vi "Whisker stim 2.vi"() -> ()   [LabVIEW 2020]
uses:
  <vilib>/MakerHub/LINX/Private/Type Defs/LINX Ref.ctl
  <vilib>/MakerHub/LINX/Private/Type Defs/Platform.ctl
  <vilib>/MakerHub/LINX/Private/Type Defs/Interface.ctl
  <vilib>/MakerHub/LINX/Private/Device/Type Defs/LINX Device Config.ctl
  <vilib>/MakerHub/LINX/Private/Device/Type Defs/TCP Config.ctl
  <vilib>/MakerHub/LINX/Private/Device/Type Defs/Channels.ctl
  <vilib>/MakerHub/LINX/Public/Peripherals/Digital/Digital Write 1 Chan.vi
  <vilib>/MakerHub/LINX/Public/Peripherals/Digital/Digital Write N Chans.vi
  <vilib>/MakerHub/LINX/Private/Local IO/LinxDigitalWrite.vi
  <vilib>/MakerHub/LINX/Public/Utilities/Check Channel.vi
  <vilib>/MakerHub/LINX/Private/Utilties/Generate Error.vi
  <vilib>/MakerHub/LINX/Public/Sensors/Motion/Servo/Servo Set Pulse Width One Channel.vi
  <vilib>/MakerHub/LINX/Public/Sensors/Motion/Servo/Servo.lvlib
  <vilib>/MakerHub/LINX/LMH-LINX.lvlib
  <vilib>/MakerHub/LINX/Private/Device/Device.lvlib
panel:
  out "Suggested P2 time (s)":dbl
  out "Seq. iteration":i32
  in  "Wheel coupled":bool
  out "Speed plot":dbl(graph)
  in  "Steps/s":u32=1000
  in  "Steps to move":dbl
  in  "Direction":bool
  in  "Stop Stepper":bool=TRUE
  in  "Start stepper":bool=TRUE caption="Start"
  in  "Direction 2":enum16{"CLW", "CCLW", "Off"}(ring)
  in  "Direction":enum16{"CLW", "CCLW", "Off"}(ring)
  in  "Speed(Steps/s) 2":u32
  in  "Speed(Steps/s)":u32
  out "Spin iteration":i32
  in  "Spin Time 2 (s)":u32
  in  "Spin n loop":i32=1
  in  "Spin Time 1 (s)":u32=5
  in  "Time(s) off":u32
  in  "Mode":enum16{"Automatic", "Manual", "Wheel"}(ring)
  out "Stop":bool
  out "Active":bool
  in  "Pole move (Pulse Width, microS)":dbl(slide)=1000.0 scale=1000.0..2000.0
  out "LINX Resource":T1
  in  "Seq loop":i32=1
  in  "Current State":string
  # "Linear Actuator"
  # "`"
  # "Stepper Motor"
  # "Auto"
  # "Manual"
  # "Wheel coupled"
  # "0 = infinite"
  # "CLW"
  # "CCLW"
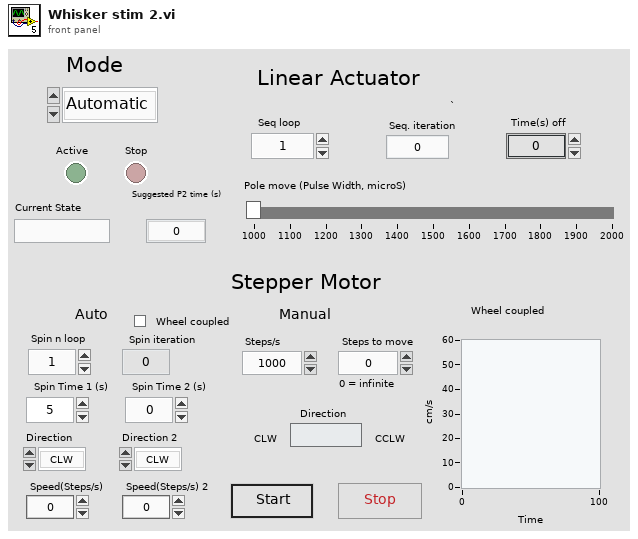
[diagram p1: front panel]
types:
  T1 = typedef "LMH-LINX.lvlib/LINX Ref.ctl" = cluster{"IO":T2, "Interface":T3, "LINX Device Config":T4}
  T2 = typedef "LMH-LINX.lvlib/Platform.ctl" = enum16{"Remote", "Local"}
  T3 = typedef "LMH-LINX.lvlib/Interface.ctl" = enum16{"Serial", "TCP"}
  T4 = typedef "LMH-LINX.lvlib/Device.lvlib/LINX Device Config.ctl" = cluster{"Interface":T3, "COM Port":refnum<visa-resource-name>, "TCP Configuration":T5, "Device Family":u8, "Device ID":u8, "Device Name":string, "TCP Ref":refnum<k5>, "Channels":T6}
  T5 = typedef "LMH-LINX.lvlib/Device.lvlib/TCP Config.ctl" = cluster{"IP Address":string, "Port":u16}
  T6 = typedef "LMH-LINX.lvlib/Channels.ctl" = cluster{"DI":u8[], "DO":u8[], "AI":u8[], "AO":u8[], "PWM":u8[], "QE":u8[], "UART":u8[], "I2C 2":u8[], "SPI":u8[], "CAN":u8[], "Servo":u8[], "AI Ref (V)":dbl, "AI Resolution (Bits)":u8, "AO Ref (V)":dbl, "AO Resolution (Bits)":u8}
  T7 = enum8{"Enabled", "Disabled", "Disabled and Grayed Out"}
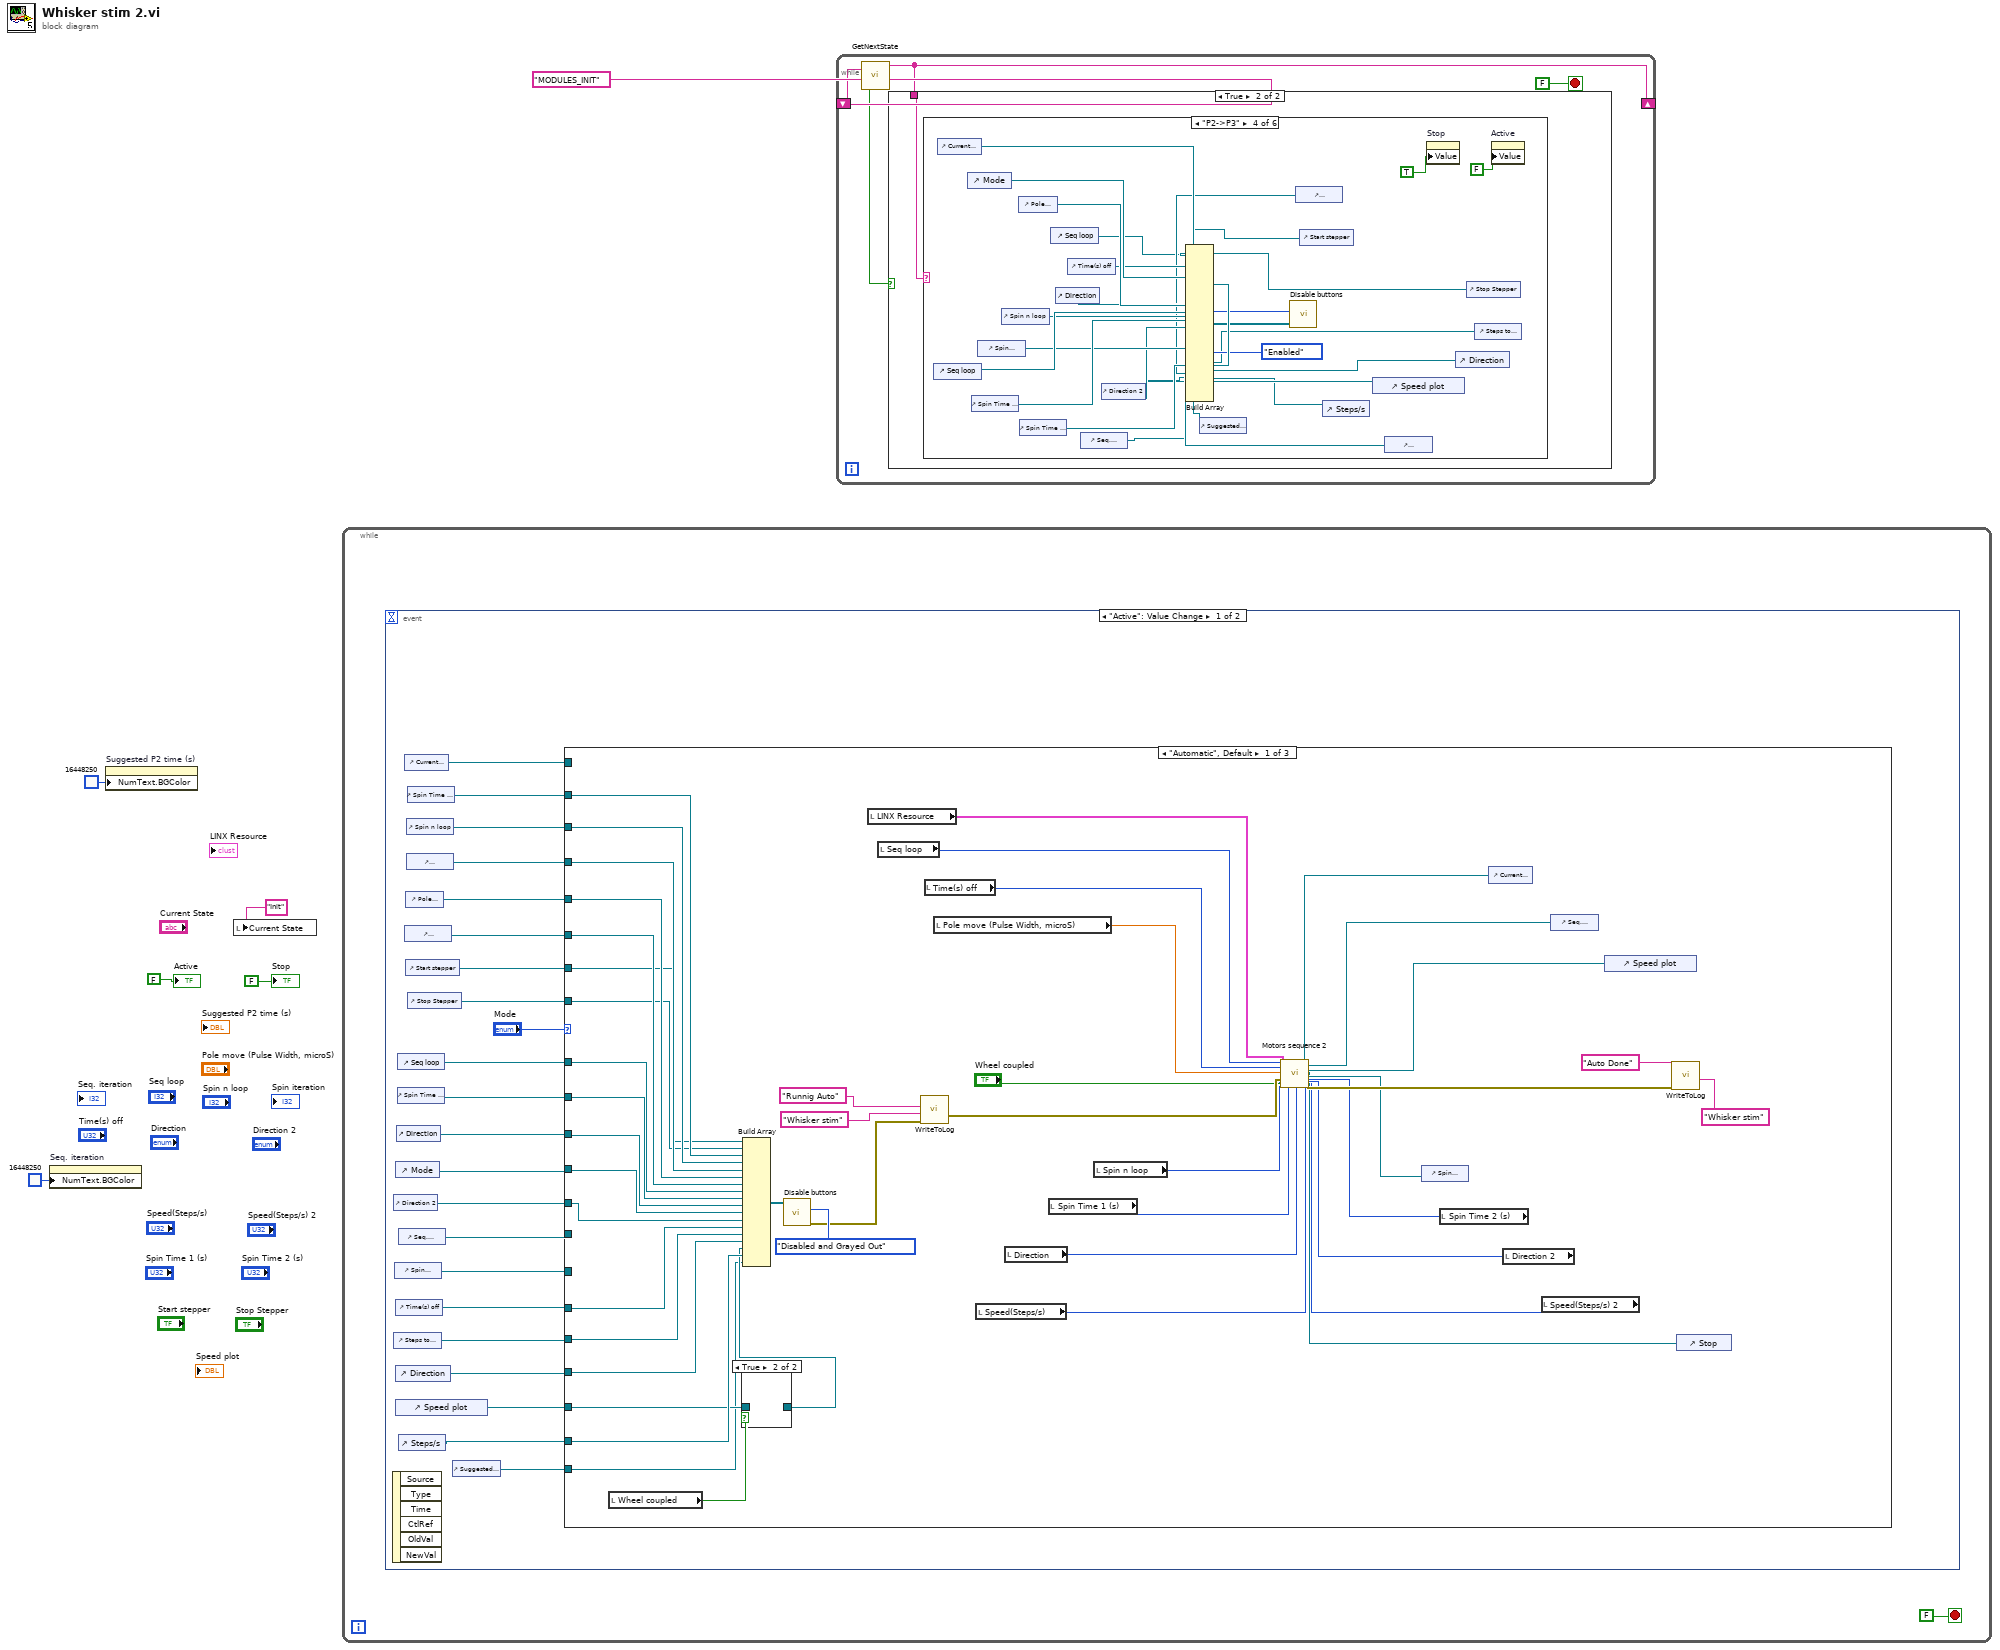
[diagram p0: block diagram]
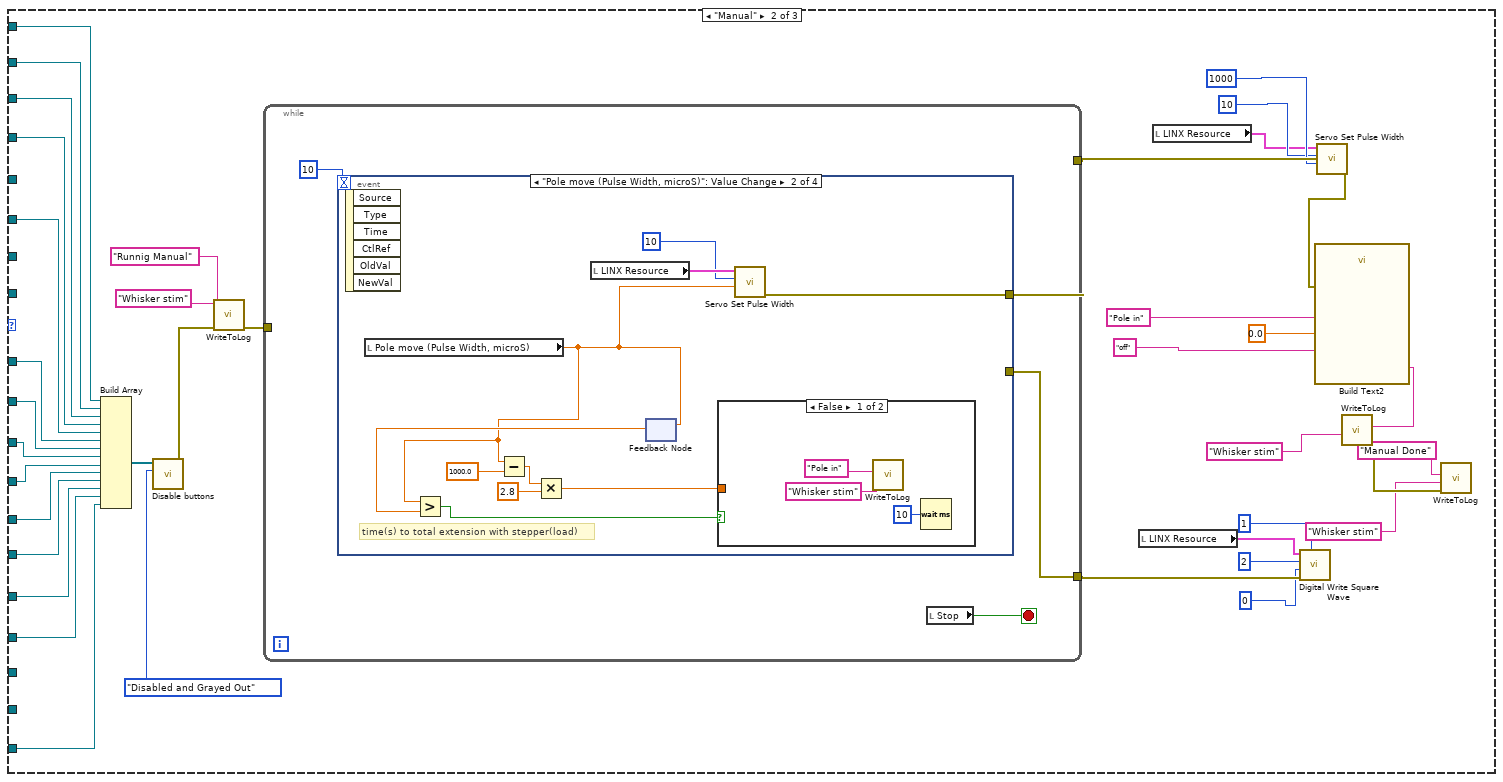
[diagram p3: hidden frame]
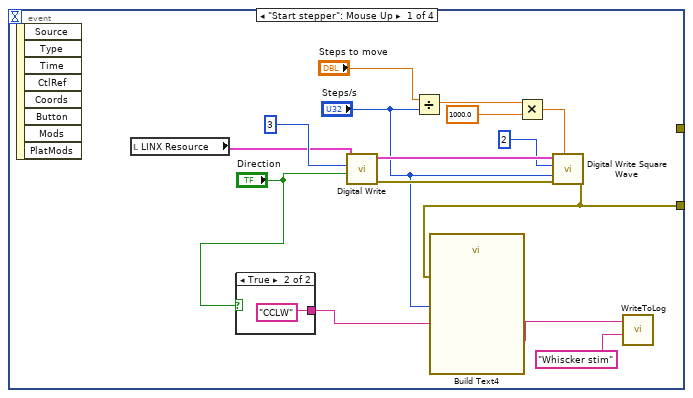
[diagram p4: hidden frame]
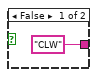
[diagram p5: hidden frame]
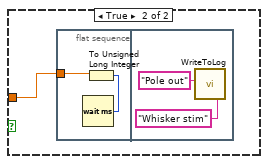
[diagram p6: hidden frame]
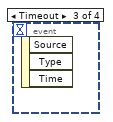
[diagram p7: hidden frame]
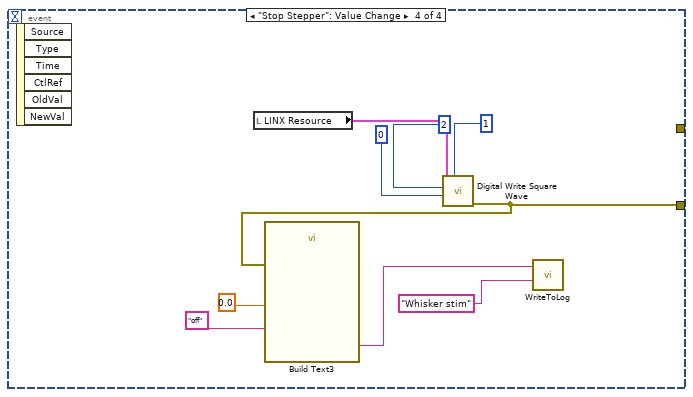
[diagram p8: hidden frame]
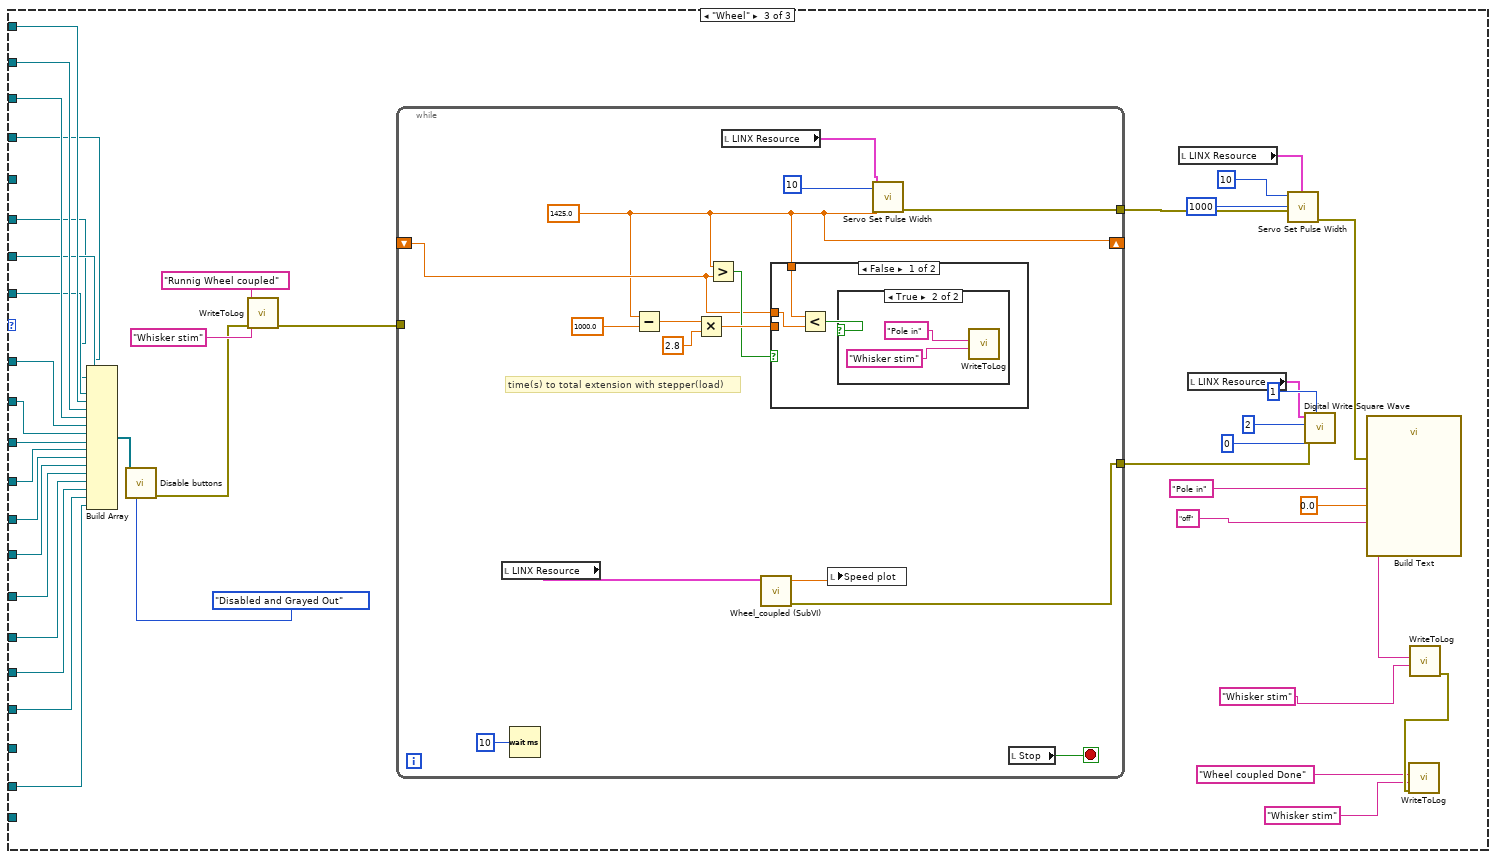
[diagram p9: hidden frame]
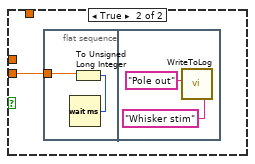
[diagram p11: hidden frame]
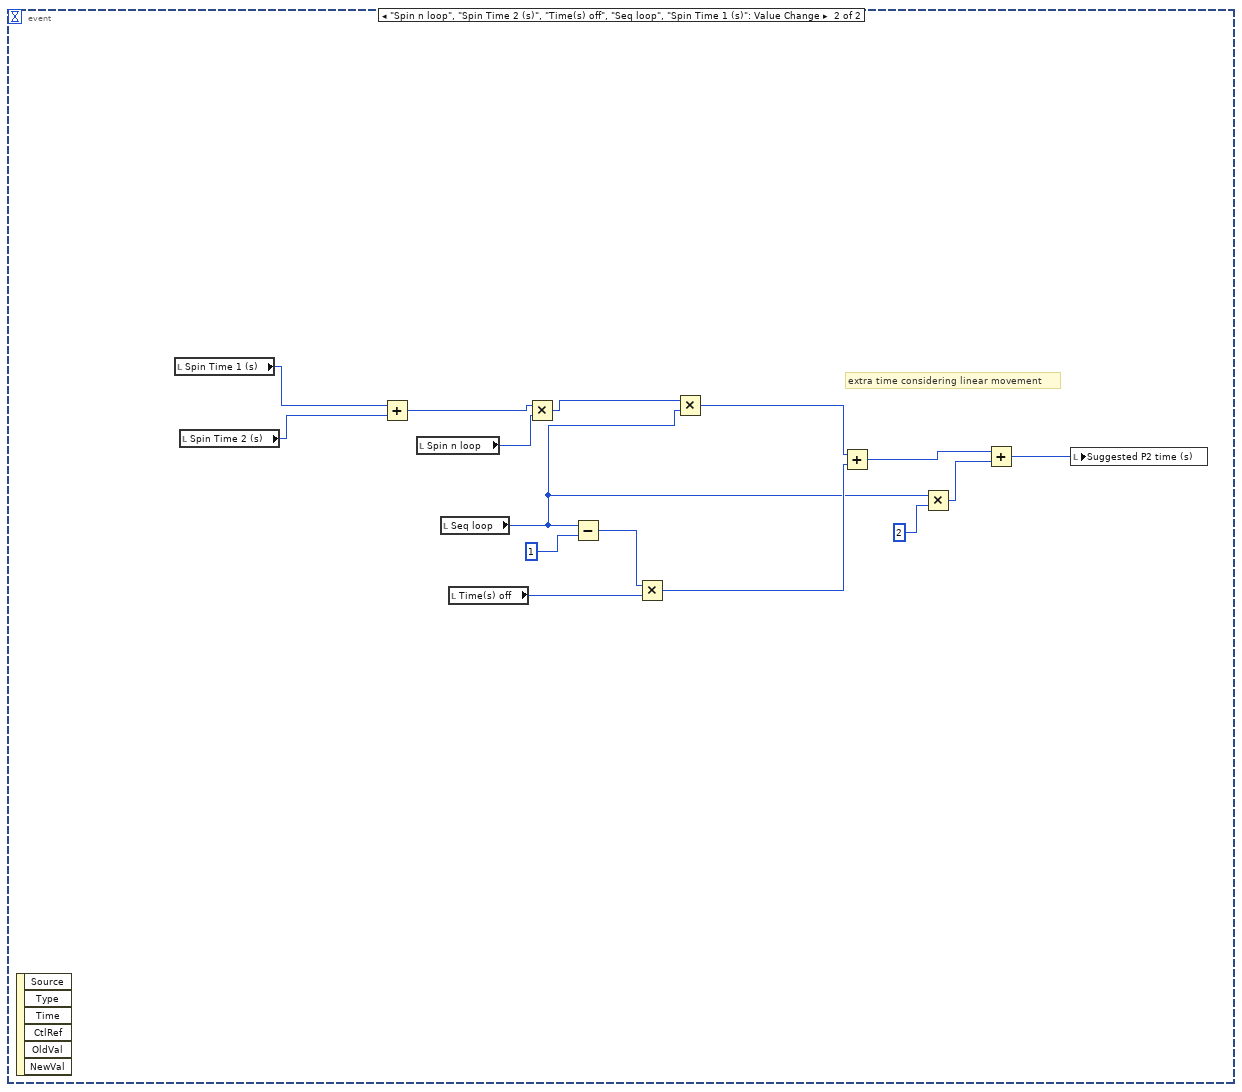
[diagram p12: hidden frame]
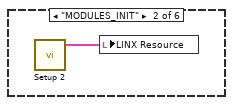
[diagram p15: hidden frame]
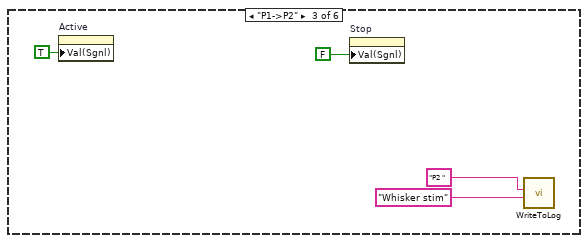
[diagram p16: hidden frame]
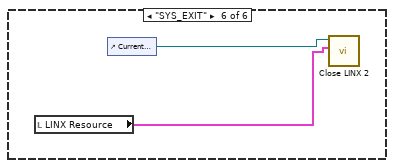
[diagram p18: hidden frame]
diagram:
  n1 = property on="Seq. iteration" class="DigNum (strict)"("NumText.BGColor"=u32 16448250 ("Numeric Text.Colors:BG Color")) -> ()  [unwired: 2 in, 2 out]
  n2 = property on="Suggested P2 time (s)" class="DigNum (strict)"("NumText.BGColor"=u32 16448250 ("Numeric Text.Text Colors:BG Color")) -> ()  [unwired: 2 in, 2 out]
  n3 = local write "Current State"("Init" ("State name")) -> ()
  n4 = while {
    stop <- FALSE stop-if-true
    n5 = event shown="[0] \"Active\": Value Change" {
      selector: _ -> [_ _]
      dyn-events: _ -> [_ _]
      timeout: _ -> [_ _]
      event "Active": Value Change {
        n6 = event-data() -> ()  [unwired: 1 in, 6 out]
        n7 = control-ref of="Direction 2"() -> (w20:refnum<vi>)
        n8 = control-ref of="Steps to move"() -> (w15:refnum<vi>)
        n9 = control-ref of="Spin iteration"() -> (w24:refnum<vi>)
        n10 = control-ref of="Mode"() -> (w25:refnum<vi>)
        n11 = control-ref of="Time(s) off"() -> (w16:refnum<vi>)
        n12 = control-ref of="Direction"() -> (w14:refnum<vi>)
        n13 = control-ref of="Speed plot"() -> (w13:refnum<vi>)
        n14 = control-ref of="Direction"() -> (w21:refnum<vi>)
        n15 = control-ref of="Seq loop"() -> (w29:refnum<vi>)
        n16 = control-ref of="Spin Time 1 (s)"() -> (w23:refnum<vi>)
        n17 = control-ref of="Seq. iteration"() -> (w9:refnum<vi>)
        n18 = control-ref of="Steps/s"() -> (w10:refnum<vi>)
        n19 = control-ref of="Current State"() -> (w22:refnum<vi>)
        n20 = control-ref of="Speed(Steps/s) 2"() -> (w18:refnum<vi>)
        n21 = control-ref of="Pole move (Pulse Width, microS)"() -> (w28:refnum<vi>)
        n22 = control-ref of="Start stepper"() -> (w12:refnum<vi>)
        n23 = control-ref of="Spin n loop"() -> (w27:refnum<vi>)
        n24 = control-ref of="Speed(Steps/s)"() -> (w19:refnum<vi>)
        n25 = control-ref of="Spin Time 2 (s)"() -> (w26:refnum<vi>)
        n26 = control-ref of="Stop Stepper"() -> (w11:refnum<vi>)
        n27 = control-ref of="Suggested P2 time (s)"() -> (w8:refnum<vi>)
        n28 = case shown="\"Automatic\", Default" "Mode" {
          tunnel: w26 -> [w73 w82 w180]
          tunnel: w27 -> [w72 w81 w179]
          tunnel: w28 -> [w70 _ _]
          tunnel: w29 -> [w68 w78 w178]
          tunnel: w21 -> [w74 w89 w176]
          tunnel: w25 -> [w75 w88 w175]
          tunnel: w20 -> [w62 w87 w174]
          tunnel: w24 -> [_ w85 w172]
          tunnel: w19 -> [w71 w80 w163]
          tunnel: w23 -> [w65 w90 w177]
          tunnel: w22 -> [_ w83 w181]
          tunnel: w18 -> [w69 w79 w164]
          tunnel: w16 -> [w67 w84 w171]
          tunnel: w9 -> [_ w86 w173]
          tunnel: w15 -> [w66 _ w170]
          tunnel: w14 -> [w64 _ w169]
          tunnel: w13 -> [w53 w77 _]
          tunnel: w10 -> [w63 _ w168]
          tunnel: w12 -> [w61 _ w166]
          tunnel: w11 -> [w60 _ w167]
          tunnel: w8 -> [w30 _ _]
          frame "Automatic", Default {
            n29 = local read "Wheel coupled"() -> (w54:bool)
            n30 = case shown="True" w54 {
              tunnel: w53 -> [w76 _]
              tunnel: [w76 _] -> w52
              frame False {
              }
              frame True {
              }
            }
            n31 = Build Array(w61, w60, w73, w72, w71, w70, w69, w68, w65, w74, w75, w62, w67, w66, w64, w52, w63, w30) -> (w59:refnum<vi>[])
            n32 = call "Disable buttons.vi"("Disabled"=T7."Disabled and Grayed Out", "Array"=w59) -> ("error out"=w55:errorcluster)  [unwired: 9 in]
            n33 = local read "LINX Resource"() -> (w47:T1)
            n34 = local read "Seq loop"() -> (w38:i32)
            n35 = call "WriteToLog.vi"("error in (no error)"=w55, "Category"="Whisker stim", "Message"="Runnig Auto") -> ("error out"=w51:errorcluster)  [unwired: 8 in]
            n36 = local read "Time(s) off"() -> (w31:u32)
            n37 = local read "Pole move (Pulse Width, microS)"() -> (w45:dbl)
            n38 = local read "Speed(Steps/s)"() -> (w44:u32)
            n39 = local read "Direction"() -> (w41:enum16{"CLW", "CCLW", "Off"})
            n40 = local read "Spin Time 1 (s)"() -> (w43:u32)
            n41 = local read "Spin n loop"() -> (w35:i32)
            n42 = control-ref of="Spin iteration"() -> (w33:refnum<vi>)
            n43 = local read "Spin Time 2 (s)"() -> (w42:u32)
            n44 = control-ref of="Current State"() -> (w46:refnum<vi>)
            n45 = local read "Direction 2"() -> (w40:enum16{"CLW", "CCLW", "Off"})
            n46 = local read "Speed(Steps/s) 2"() -> (w36:u32)
            n47 = control-ref of="Seq. iteration"() -> (w34:refnum<vi>)
            n48 = control-ref of="Speed plot"() -> (w37:refnum<vi>)
            n49 = control-ref of="Stop"() -> (w32:refnum<vi>)
            n50 = call "Motors sequence 2.vi"("LINX Resource"=w47, "Current State"=w46, "Pole move(microS)"=w45, "Speed(Steps/s)"=w44, "Error In"=w51, "Wheel"="Wheel coupled", "Spin time/Rest(1)"=w43, "Spin n loops"=w35, "Spin time(2)"=w42, "Speed(Steps/s) 2"=w36, "Direction"=w41, "Pole ms to wait off"=w31, "Direction 2"=w40, "Seq. iteration 2"=w34, "Stop"=w32, "Speed plot 2"=w37, "Seq. loop"=w38, "Spin iteration 2"=w33) -> ("error out"=w48:errorcluster)  [unwired: 8 in, 1 out]
            n51 = call "WriteToLog.vi"("error in (no error)"=w48, "Category"="Whisker stim", "Message"="Auto Done") -> ()  [unwired: 8 in, 1 out]
          }
          frame "Manual" {
            n52 = Build Array(w83, w82, w81, w80, w79, w78, w90, w89, w88, w87, w86, w85, w84, w77) -> (w91:refnum<vi>[])
            n53 = call "Disable buttons.vi"("Disabled"=T7."Disabled and Grayed Out", "Array"=w91) -> ("error out"=w97:errorcluster)  [unwired: 9 in]
            n54 = call "WriteToLog.vi"("error in (no error)"=w97, "Category"="Whisker stim", "Message"="Runnig Manual") -> ("error out"=w96:errorcluster)  [unwired: 8 in]
            n55 = while {
              tunnel: [w116] -> w113
              tunnel: [w115] -> w110
              tunnel: w96 -> [_]
              stop <- w118 stop-if-true
              n56 = event shown="[1] \"Pole move (Pulse Width, microS)\": Value Change" {
                selector: _ -> [_ _ _ _]
                dyn-events: _ -> [_ _ _ _]
                timeout: 10 -> [_ _ _ _]
                tunnel: [_ w143 _ _] -> w116
                tunnel: [w122 _ _ w154] -> w115
                event "Start stepper": Mouse Up {
                  n57 = event-data() -> ()  [unwired: 1 in, 8 out]
                  n58 = local read "LINX Resource"() -> (w126:T1)
                  n59 = case shown="True" "Direction" {
                    tunnel: ["CLW" "CCLW"] -> w120
                    frame False {
                    }
                    frame True {
                    }
                  }
                  n60 = call-poly <vilib>:"Digital Write.vi"("Output Value"="Direction", "DO Channel"=u8 3, "LINX Resource"=w126) -> ("Error Out"=w123:errorcluster, "LINX Resource"=w130:T1)  [unwired: 7 in]
                  n61 = Divide(x="Steps to move", y="Steps/s") -> (x/y=w128:dbl)
                  n62 = Multiply(x=w128, y=1000.0) -> (x*y=w132:dbl)
                  n63 = call <vilib>:"Digital Write Square Wave.vi"("Duration (ms)"=w132, "Error In"=w123, "Frequency (Hz)"="Steps/s", "Channel"=u8 2, "LINX Resource"=w130) -> ("Error Out"=w122:errorcluster)  [unwired: 5 in, 1 out]
                  n64 = call "Build Text4"("speed"="Steps/s", "spinmode"=w120, "error in (no error)"=w122) -> ("Result"=w124:string)  [unwired: 11 in, 1 out]
                  n65 = call "WriteToLog.vi"("Category"="Whiscker stim", "Message"=w124) -> ()  [unwired: 9 in, 1 out]
                }
                event "Pole move (Pulse Width, microS)": Value Change {
                  # "time(s) to total extension with stepper(load)"
                  n66 = event-data() -> ()  [unwired: 1 in, 6 out]
                  n67 = local read "Pole move (Pulse Width, microS)"() -> (w136:dbl)
                  n68 = Subtract(x=w136, y=1000.0) -> (x-y=w142:dbl)
                  n69 = Multiply(x=w142, y=2.8) -> (x*y=w139:dbl)
                  n70 = local read "LINX Resource"() -> (w145:T1)
                  n71 = feedback #1() -> (w137:dbl)  [unwired: 1 in]
                  n72 = Greater?(x=w136, y=w137) -> (0:w138:bool)
                  n73 = feedback-in #1(w136) -> ()
                  n74 = case shown="False" w138 {
                    tunnel: w139 -> [_ w149]
                    frame False {
                      n75 = call "WriteToLog.vi"("Category"="Whisker stim", "Message"="Pole in") -> ()  [unwired: 9 in, 1 out]
                      n76 = Wait (ms)(milliseconds to wait=u32 10) -> ()  [unwired: 1 out]
                    }
                    frame True {
                      n77 = flat-sequence {
                        tunnel: w149 -> [w150]
                        frame #0 {
                          n78 = To Unsigned Long Integer(number=w150) -> (unsigned 32bit integer=w151:u32)
                          n79 = Wait (ms)(milliseconds to wait=w151) -> ()  [unwired: 1 out]
                        }
                        frame #1 {
                          n80 = call "WriteToLog.vi"("Category"="Whisker stim", "Message"="Pole out") -> ()  [unwired: 9 in, 1 out]
                        }
                      }
                    }
                  }
                  n81 = call-poly <vilib>:"Servo Set Pulse Width.vi"("Pulse Width (uS)"=w136, "Servo Channel"=u8 10, "LINX Resource"=w145) -> ("Error Out"=w143:errorcluster)  [unwired: 7 in, 1 out]
                }
                event Timeout {
                  n82 = event-data() -> ()  [unwired: 1 in, 3 out]
                }
                event "Stop Stepper": Value Change {
                  n83 = event-data() -> ()  [unwired: 1 in, 6 out]
                  n84 = local read "LINX Resource"() -> (w159:T1)
                  n85 = call <vilib>:"Digital Write Square Wave.vi"("Duration (ms)"=u32 1, "Frequency (Hz)"=u32 0, "Channel"=u8 2, "LINX Resource"=w159) -> ("Error Out"=w154:errorcluster)  [unwired: 6 in, 1 out]
                  n86 = call "Build Text3"("speed"=0.0, "spinmode"="off", "error in (no error)"=w154) -> ("Result"=w156:string)  [unwired: 11 in, 1 out]
                  n87 = call "WriteToLog.vi"("Category"="Whisker stim", "Message"=w156) -> ()  [unwired: 9 in, 1 out]
                }
              }
              n88 = local read "Stop"() -> (w118:bool)
            }
            n89 = local read "LINX Resource"() -> (w105:T1)
            n90 = local read "LINX Resource"() -> (w106:T1)
            n91 = call <vilib>:"Digital Write Square Wave.vi"("Duration (ms)"=u32 1, "Error In"=w110, "Frequency (Hz)"=u32 0, "Channel"=u8 2, "LINX Resource"=w105) -> ()  [unwired: 5 in, 2 out]
            n92 = call-poly <vilib>:"Servo Set Pulse Width.vi"("Error In"=w113, "Pulse Width (uS)"=u16 1000, "Servo Channel"=u8 10, "LINX Resource"=w106) -> ("Error Out"=w98:errorcluster)  [unwired: 6 in, 1 out]
            n93 = call "Build Text2"("speed"=0.0, "spinmode"="off", "step"="Pole in", "error in (no error)"=w98) -> ("Result"=w102:string)  [unwired: 10 in, 1 out]
            n94 = call "WriteToLog.vi"("Category"="Whisker stim", "Message"=w102) -> ("error out"=w94:errorcluster)  [unwired: 9 in]
            n95 = call "WriteToLog.vi"("error in (no error)"=w94, "Category"="Whisker stim", "Message"="Manual Done") -> ()  [unwired: 8 in, 1 out]
          }
          frame "Wheel" {
            n96 = Build Array(w163, w164, w166, w167, w181, w180, w179, w178, w177, w176, w175, w174, w173, w172, w171, w170, w169, w168) -> (w165:refnum<vi>[])
            n97 = call "Disable buttons.vi"("Disabled"=T7."Disabled and Grayed Out", "Array"=w165) -> ("error out"=w185:errorcluster)  [unwired: 9 in]
            n98 = call "WriteToLog.vi"("error in (no error)"=w185, "Category"="Whisker stim", "Message"="Runnig Wheel coupled") -> ("error out"=w186:errorcluster)  [unwired: 8 in]
            n99 = while {
              tunnel: [w217] -> w204
              tunnel: [w213] -> w197
              shift-right: [w206] -> _
              shift-left: _ -> [w207]
              tunnel: w186 -> [_]
              stop <- w219 stop-if-true
              w206 = 1425.0 ("Pole move (Pulse Width, microS)")
              # "time(s) to total extension with stepper(load)"
              n100 = local read "LINX Resource"() -> (w218:T1)
              n101 = Wait (ms)(milliseconds to wait=u32 10) -> ()  [unwired: 1 out]
              n102 = Subtract(x=w206, y=1000.0) -> (x-y=w211:dbl)
              n103 = Multiply(x=w211, y=2.8) -> (x*y=w209:dbl)
              n104 = Greater?(x=w206, y=w207) -> (0:w208:bool)
              n105 = local read "LINX Resource"() -> (w215:T1)
              n106 = call "Wheel_coupled (SubVI).vi"("LINX Resource"=w218) -> ("error out"=w217:errorcluster, "Speed plot"=w205:dbl)  [unwired: 9 in]
              n107 = case shown="False" w208 {
                tunnel: w209 -> [_ w225]
                tunnel: w206 -> [w222 _]
                tunnel: w207 -> [w221 _]
                frame False {
                  n108 = Less?(x=w222, y=w221) -> (x < y?=w220:bool)
                  n109 = case shown="True" w220 {
                    frame False {
                    }
                    frame True {
                      n110 = call "WriteToLog.vi"("Category"="Whisker stim", "Message"="Pole in") -> ()  [unwired: 9 in, 1 out]
                    }
                  }
                }
                frame True {
                  n111 = flat-sequence {
                    tunnel: w225 -> [w226]
                    frame #0 {
                      n112 = To Unsigned Long Integer(number=w226) -> (unsigned 32bit integer=w227:u32)
                      n113 = Wait (ms)(milliseconds to wait=w227) -> ()  [unwired: 1 out]
                    }
                    frame #1 {
                      n114 = call "WriteToLog.vi"("Category"="Whisker stim", "Message"="Pole out") -> ()  [unwired: 9 in, 1 out]
                    }
                  }
                }
              }
              n115 = local write "Speed plot"(w205) -> ()
              n116 = call-poly <vilib>:"Servo Set Pulse Width.vi"("Pulse Width (uS)"=w206, "Servo Channel"=u8 10, "LINX Resource"=w215) -> ("Error Out"=w213:errorcluster)  [unwired: 7 in, 1 out]
              n117 = local read "Stop"() -> (w219:bool)
            }
            n118 = local read "LINX Resource"() -> (w198:T1)
            n119 = local read "LINX Resource"() -> (w201:T1)
            n120 = call-poly <vilib>:"Servo Set Pulse Width.vi"("Error In"=w197, "Pulse Width (uS)"=u16 1000, "Servo Channel"=u8 10, "LINX Resource"=w198) -> ("Error Out"=w188:errorcluster)  [unwired: 6 in, 1 out]
            n121 = call <vilib>:"Digital Write Square Wave.vi"("Duration (ms)"=u32 1, "Error In"=w204, "Frequency (Hz)"=u32 0, "Channel"=u8 2, "LINX Resource"=w201) -> ()  [unwired: 5 in, 2 out]
            n122 = call "Build Text"("speed"=0.0, "spinmode"="off", "step"="Pole in", "error in (no error)"=w188) -> ("Result"=w190:string)  [unwired: 10 in, 1 out]
            n123 = call "WriteToLog.vi"("Category"="Whisker stim", "Message"=w190) -> ("error out"=w184:errorcluster)  [unwired: 9 in]
            n124 = call "WriteToLog.vi"("error in (no error)"=w184, "Category"="Whisker stim", "Message"="Wheel coupled Done") -> ()  [unwired: 8 in, 1 out]
          }
        }
      }
      event "Spin n loop", "Spin Time 2 (s)", "Time(s) off", "Seq loop", "Spin Time 1 (s)": Value Change {
        # "extra time considering linear movement"
        n125 = event-data() -> ()  [unwired: 1 in, 6 out]
        n126 = local read "Spin Time 1 (s)"() -> (w243:u32)
        n127 = local read "Spin Time 2 (s)"() -> (w244:u32)
        n128 = Add(x=w243, y=w244) -> (x+y=w242:u32)
        n129 = local read "Spin n loop"() -> (w241:i32)
        n130 = local read "Seq loop"() -> (w233:i32)
        n131 = local read "Time(s) off"() -> (w239:u32)
        n132 = Multiply(x=w242, y=w241) -> (x*y=w240:u32)
        n133 = Subtract(x=w233, y=1) -> (x-y=w237:i32)
        n134 = Multiply(x=w237, y=w239) -> (x*y=w235:u32)
        n135 = Multiply(x=w240, y=w233) -> (x*y=w236:u32)
        n136 = Add(x=w236, y=w235) -> (x+y=w234:u32)
        n137 = Multiply(x=w233, y=2) -> (x*y=w231:i32)
        n138 = Add(x=w234, y=w231) -> (x+y=w230:u32)
        n139 = local write "Suggested P2 time (s)"(w230) -> ()
      }
    }
  }
  n140 = while {
    shift-right: [w245] -> _
    shift-left: "MODULES_INIT" ("Next state") -> [w247]
    stop <- FALSE stop-if-true
    n141 = call "GetNextState.vi"("Current state"=w247) -> ("State has changed?"=w246:bool, "Next state"=w245:string)  [unwired: 9 in]
    n142 = case shown="True" w246 {
      tunnel: w245 -> [_ w249]
      frame False {
      }
      frame True {
        n143 = case shown="\"P2->P3\"" w249 {
          frame "False", Default {
          }
          frame "MODULES_INIT" {
            n144 = call "Setup 2.vi"() -> ("LINX Resource"=w250:T1)  [unwired: 10 in, 1 out]
            n145 = local write "LINX Resource"(w250) -> ()
          }
          frame "P1->P2" {
            n146 = property on="Active" class="Bool (strict)"("Val(Sgnl)"=TRUE ("Value (Signaling)")) -> ()  [unwired: 2 in, 2 out]
            n147 = property on="Stop" class="Bool (strict)"("Val(Sgnl)"=FALSE ("Value (Signaling)")) -> ()  [unwired: 2 in, 2 out]
            n148 = call "WriteToLog.vi"("Category"="Whisker stim", "Message"="P2 ") -> ()  [unwired: 9 in, 1 out]
          }
          frame "P2->P3" {
            n149 = control-ref of="Seq loop"() -> (w277:refnum<vi>)
            n150 = control-ref of="Current State"() -> (w268:refnum<vi>)
            n151 = control-ref of="Mode"() -> (w271:refnum<vi>)
            n152 = control-ref of="Spin Time 1 (s)"() -> (w278:refnum<vi>)
            n153 = control-ref of="Spin iteration"() -> (w270:refnum<vi>)
            n154 = control-ref of="Spin n loop"() -> (w275:refnum<vi>)
            n155 = control-ref of="Pole move (Pulse Width, microS)"() -> (w276:refnum<vi>)
            n156 = control-ref of="Spin Time 2 (s)"() -> (w274:refnum<vi>)
            n157 = control-ref of="Seq loop"() -> (w257:refnum<vi>)
            n158 = control-ref of="Direction"() -> (w267:refnum<vi>)
            n159 = control-ref of="Time(s) off"() -> (w269:refnum<vi>)
            n160 = control-ref of="Seq. iteration"() -> (w256:refnum<vi>)
            n161 = control-ref of="Direction 2"() -> (w266:refnum<vi>)
            n162 = control-ref of="Suggested P2 time (s)"() -> (w255:refnum<vi>)
            n163 = control-ref of="Speed(Steps/s)"() -> (w265:refnum<vi>)
            n164 = control-ref of="Start stepper"() -> (w259:refnum<vi>)
            n165 = control-ref of="Steps/s"() -> (w260:refnum<vi>)
            n166 = control-ref of="Speed plot"() -> (w261:refnum<vi>)
            n167 = control-ref of="Speed(Steps/s) 2"() -> (w264:refnum<vi>)
            n168 = property on="Stop" class="Bool (strict)"("Value"=TRUE ("Stop")) -> ()  [unwired: 2 in, 2 out]
            n169 = control-ref of="Direction"() -> (w262:refnum<vi>)
            n170 = control-ref of="Stop Stepper"() -> (w258:refnum<vi>)
            n171 = control-ref of="Steps to move"() -> (w263:refnum<vi>)
            n172 = Build Array(w259, w258, w268, w269, w271, w274, w275, w267, w276, w277, w278, w266, w265, w257, w270, w264, w263, w262, w261, w260, w256, w255) -> (w273:refnum<vi>[])
            n173 = call "Disable buttons.vi"("Disabled"=T7."Enabled", "Array"=w273) -> ()  [unwired: 9 in, 1 out]
            n174 = property on="Active" class="Bool (strict)"("Value"=FALSE ("Adquire")) -> ()  [unwired: 2 in, 2 out]
          }
          frame "P3" {
          }
          frame "SYS_EXIT" {
            n175 = local read "LINX Resource"() -> (w281:T1)
            n176 = control-ref of="Current State"() -> (w282:refnum<vi>)
            n177 = call "Close LINX 2.vi"("LINX Resource"=w281, "String in"=w282) -> ()  [unwired: 10 in]
          }
        }
      }
    }
  }
  "Active" <- FALSE ("Adquire")
  "Stop" <- FALSE ("Stop")
